vi "Configure File Extension.vi"(8 "Error In":errorcluster, 11 "File Extension":string="csv") -> (0 "Error Out":errorcluster)   [LabVIEW 2015, in "Logger.lvlib"]
doc: "Changes the default log file extension. The default is \"csv\"."
uses:
  Logger.lvlib
  Private/File/Action.ctl
  Private/File/File.lvlib
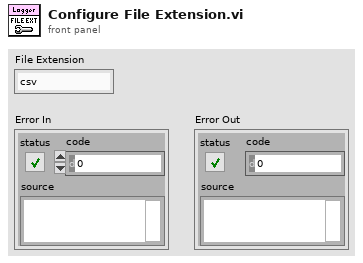
[diagram p1: front panel]
types:
  T1 = typedef "Logger.lvlib/File.lvlib/Action.ctl" = enum16{"Initialize", "Set Maximum File Size", "Set Maximum File Count", "Set Root Folder", "Set Enable Calendar Folder Tree", "Set File Extension", "Start", "Write", "Stop", "Shutdown"}
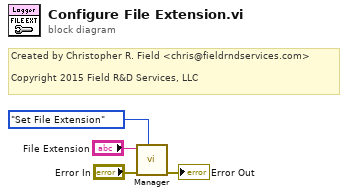
[diagram p0: block diagram]
diagram:
  # "Created by Christopher R. Field <chris@fieldrndservices.com>\n\nCopyright 2015 Field R&D Services, LLC"
  n1 = call "Manager.vi"("Action"=Action."Set File Extension", "Error In"="Error In", "Set Value"="File Extension") -> ("Error Out"=→"Error Out":errorcluster)  [unwired: 8 in]
